vi "action.vi"(0 "HGF_FGV_Append":refnum<class "HGF_FGV_Clear.lvclass">, 2 "Objects":refnum<class>[](array[class]), 5 "error in (no error)":errorcluster) -> (14 "dup HGF_FGV_Append":refnum<class "HGF_FGV_Clear.lvclass">, 16 "dup Objects":refnum<class>[](array[class]), 19 "error out":errorcluster)   [LabVIEW 2012, in "HGF_FGV.lvlib" / "HGF_FGV_Clear.lvclass"]
doc: "Clear object array."
uses:
  HGF_FGV_Clear.lvclass
  HGF_FGV_Clear.lvclass/HGF_FGV_Clear.ctl
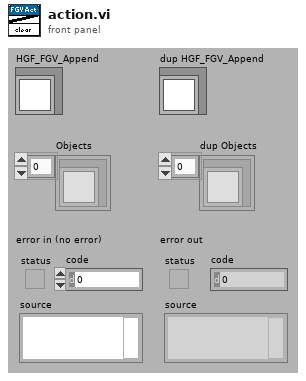
[diagram p1: front panel]
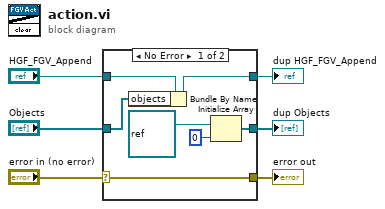
[diagram p0: block diagram]
diagram:
  n1 = case shown="No Error" "error in (no error)" {
    selector: "error in (no error)" -> [w13 w16]
    tunnel: [w13 w16] -> w5
    tunnel: [w11 w15] -> w3
    tunnel: "HGF_FGV_Append" -> [w12 w15]
    tunnel: [w9 w14] -> w2
    tunnel: "Objects" -> [w10 w14]
    frame No Error {
      n2 = Bundle By Name(cluster=w12, "objects"=w10) -> (w11:refnum<class "HGF_FGV_Clear.lvclass">)
      n3 = Initialize Array(refnum<class> refnum ("LabVIEW Object"), 0 ("dimension size")) -> (w9:refnum<class>[])
    }
    frame Error {
    }
  }
  "error out" <- w5
  "dup HGF_FGV_Append" <- w3
  "dup Objects" <- w2
